vi "Teleop.vi"(10 "Match Info":T2={"Autonomous Elapsed Seconds"=0.0, "TeleOp Elapsed Seconds"=0.0, "Disabled Elapsed Seconds"=0.0, "Visited Autonomous"=FALSE, "Visited TeleOp"=FALSE, "Visited Disabled"=FALSE, "Autonomous Settings"={"Autonomous Style"=enum."Independent", "VI Refnum"=refnum}}, 11 "Call Context":T3) -> ()   [LabVIEW 2015]
doc: "This VI is called for each TeleOp packet received from the DS where the robot is not disabled. It is often used to read from the joysticks and update I/O or to update setpoints for timed control loops. It should complete and return within 20 milliseconds or it may miss DS packets."
uses:
  <vilib>/Rock Robotics/WPI/DriverStation/WPI_DriverStationDerivedRobotMode.ctl
  <vilib>/Rock Robotics/WPI/DriverStation/WPI_DriverStationMatch Info.ctl
  <vilib>/Rock Robotics/WPI/Utilities/WPI_GetSetVariantRefNum.vi
  <vilib>/Rock Robotics/Network Tables/SD Write Boolean Array.vi
  <vilib>/Rock Robotics/Network Tables/SD Read Boolean.vi
  <vilib>/Rock Robotics/Network Tables/SD Read Number.vi
  Robot Global Data.vi
  <vilib>/addons/control/pid/pid.llb/PID (DBL).vi
  <vilib>/Rock Robotics/WPI/RobotDrive/WPI_RobotDriveMecanumDrive_Cartesian.vi
  <vilib>/addons/control/pid/NI_PID_pid.lvlib
panel:
  in  "UseGyro?":bool
  out "Gyro":T1(graph)
  out "Rotation Input":dbl(graph)
  out "Sample Slider 0":dbl(slide) scale=0.0..5.0
  out "Sample Boolean 1":bool
  out "Sample Boolean 0":bool
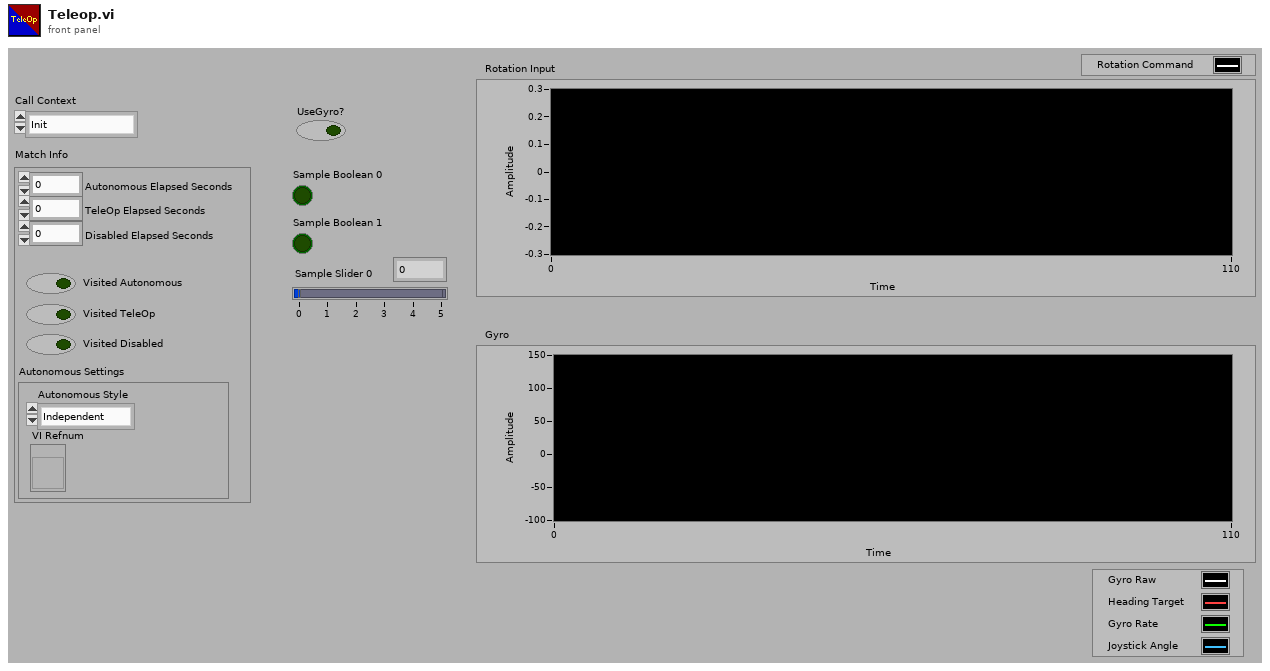
[diagram p1: front panel]
types:
  T1 = cluster{"Angle":dbl, "Heading":dbl, "Angular Rate":dbl, dbl}
  T2 = typedef "WPI_DriverStationMatch Info.ctl" = cluster{"Autonomous Elapsed Seconds":dbl, "TeleOp Elapsed Seconds":dbl, "Disabled Elapsed Seconds":dbl, "Visited Autonomous":bool, "Visited TeleOp":bool, "Visited Disabled":bool, "Autonomous Settings":cluster{"Autonomous Style":enum16{"Iterative", "Independent"}, "VI Refnum":refnum<vi>}}
  T3 = typedef "WPI_DriverStationDerivedRobotMode.ctl" = enum16{"Init", "Execute", "Stop"}
  T4 = cluster{"proportional gain (Kc)":dbl, "integral time (Ti, min)":dbl, "derivative time (Td, min)":dbl}
  T5 = typedef "WPI_JoystickDevRef.ctl" = cluster{"Device":T6}
  T6 = typedef "WPI_JoystickDeviceEnum.ctl" = enum16{"USB 0", "USB 1", "USB 2", "USB 3", "USB 4", "USB 5"}
  T7 = cluster{"Axes[0]":dbl, "Axes[1]":dbl, "Axes[2]":dbl, "Axes[3]":dbl, "Axes[4]":dbl, "Axes[5]":dbl, "Axes[6]":dbl, "Axes[7]":dbl, "Axes[8]":dbl}
  T8 = cluster{"Buttons[0]":bool, "Buttons[1]":bool, "Buttons[2]":bool, "Buttons[3]":bool, "Buttons[4]":bool, "Buttons[5]":bool, "Buttons[6]":bool, "Buttons[7]":bool, "Buttons[8]":bool}
  T9 = enum16{"CW_Fast", "CW_Slow", "CCW_Fast", "CCW_Slow", "Straight", "WaitingForStraight", "Rotate_Move"}
  T10 = cluster{"GyroHeading":dbl, "Heading":dbl, "GyroRate":dbl, dbl}
  T11 = typedef "WPI_RobotDriveDevRef.ctl" = cluster{"DevStatus":errorcluster, "Motors[]":T12[], "Square Inputs":bool, "Max Output":dbl}
  T12 = typedef "WPI_MotorControlDeviceRef.ctl" = cluster{"DeviceStatus":errorcluster, "Type":T13, "PWM":cluster{"PWM Channel":T14, "DeadBand":T15}, "CAN":cluster{"Device Number":u8, "Control Mode":T16, "Semaphore":T17, "Max Vout":dbl, "TalonSRX Control Mode":T18}, "Invert":bool}
  T13 = typedef "WPI_MotorControlType.ctl" = enum16{"PWM", "CAN", "CANTalonSRX"}
  T14 = typedef "FPGA_DIOPWMChannel.ctl" = enum8{"PWM 0", "PWM 1", "PWM 2", "PWM 3", "PWM 4", "PWM 5", "PWM 6", "PWM 7", "PWM 8", "PWM 9", "PWM MXP 0", "PWM MXP 1", "PWM MXP 2", "PWM MXP 3", "PWM MXP 4", "PWM MXP 5", "PWM MXP 6", "PWM MXP 7", "PWM MXP 8", "PWM MXP 9", "Invalid"}
  T15 = typedef "WPI_PWMDeadband.ctl" = cluster{"Name":string, "maxPositivePwm":i32, "minPositivePwm":i32, "centerPwm":i32, "maxNegativePwm":i32, "minNegativePwm":i32, "angularRange":u16}
  T16 = typedef "WPI_CANJaguar_ControlMode.ctl" = enum8{"Percent VBus", "Current", "Speed", "Position", "Voltage"}
  T17 = typedef "Semaphore RefNum" = refnum<k1>
  T18 = typedef "WPI_CANTalonSRX_APIControlMode.ctl" = enum8{"Percent VBus", "Speed", "Position", "Slave", "Unchanged / Invalid", "Voltage Compensation", "Current"}
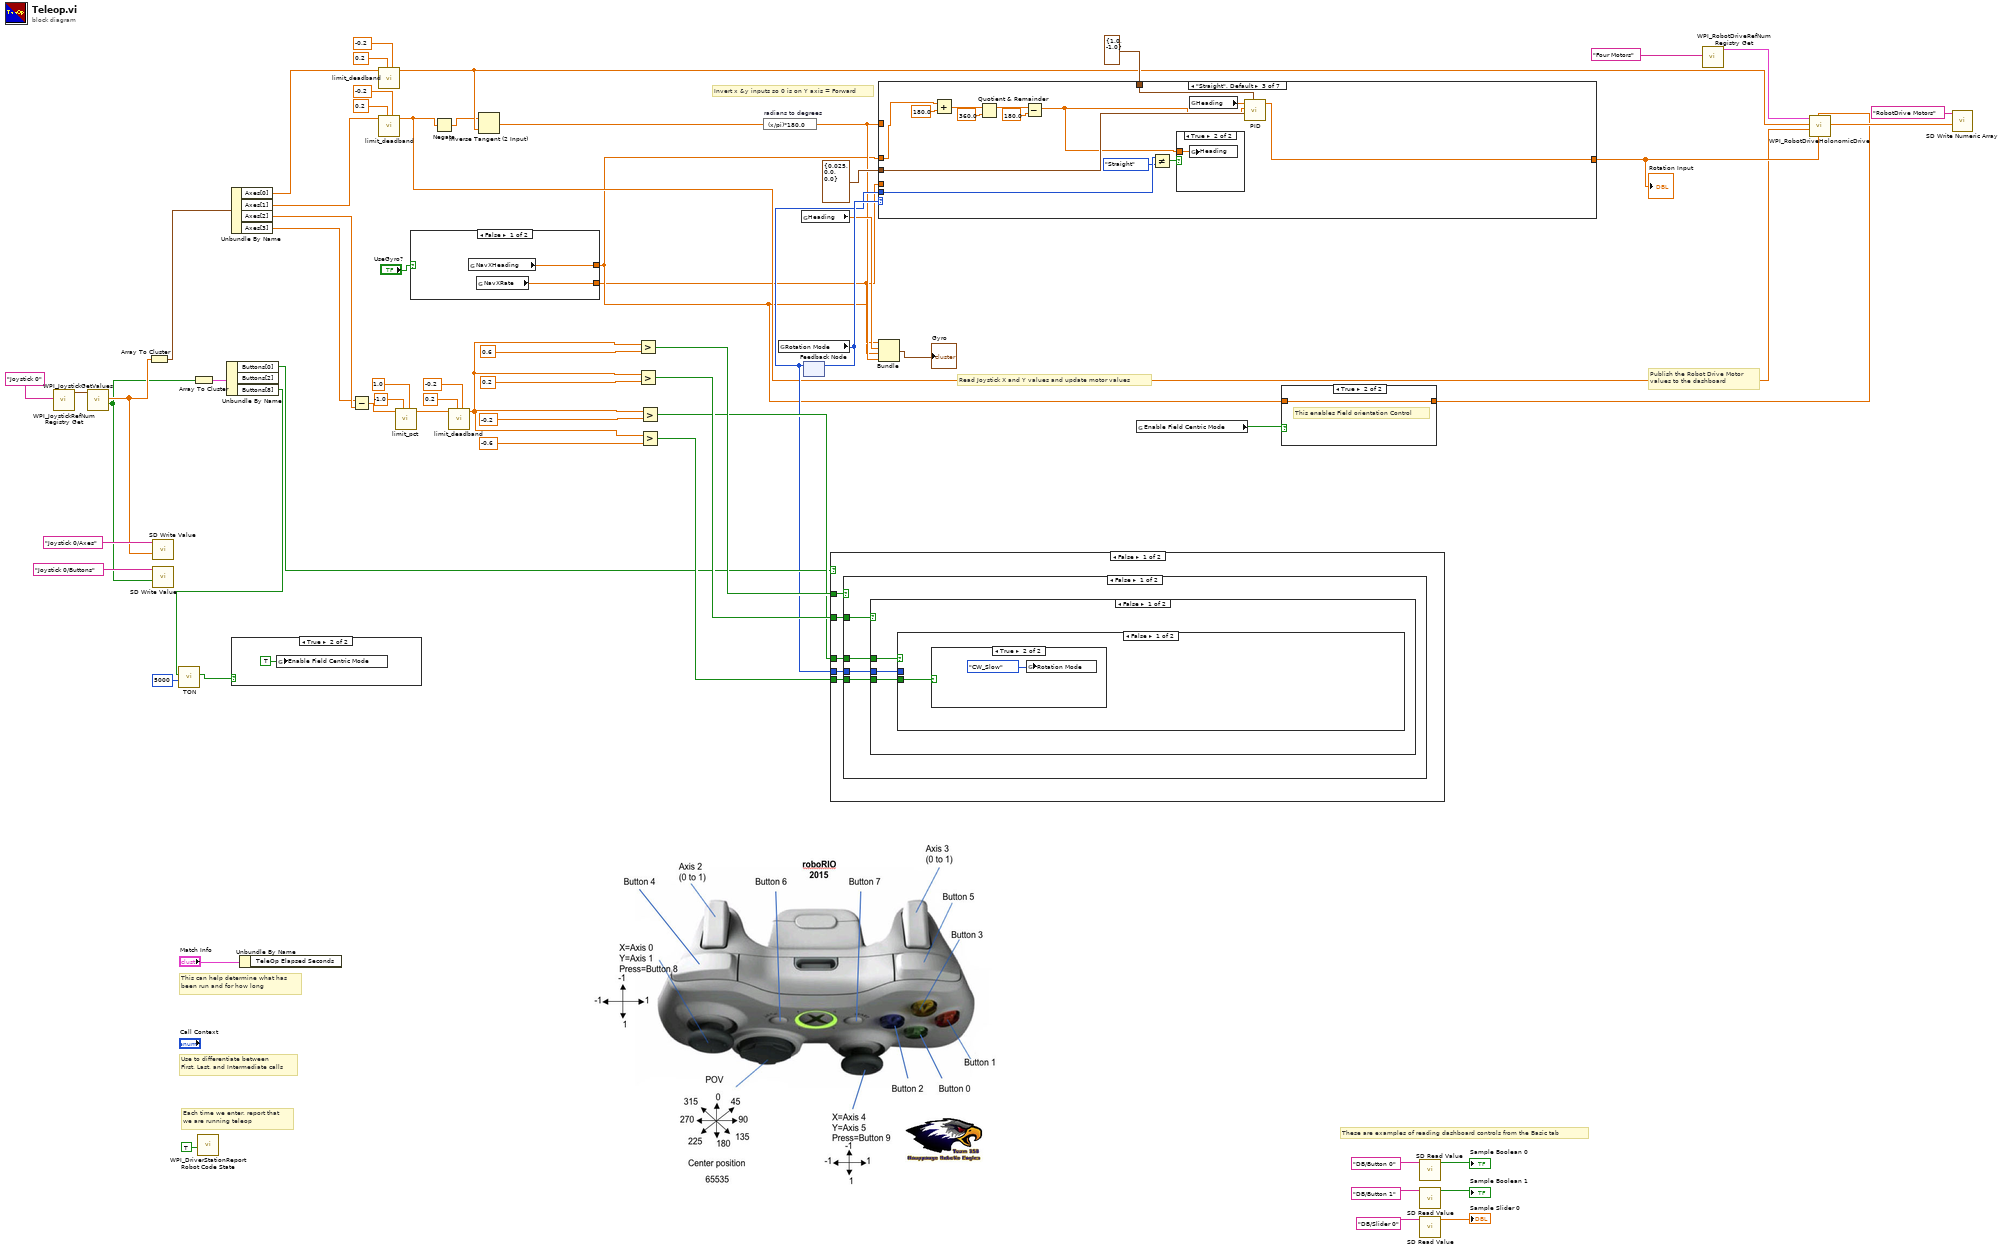
[diagram p0: block diagram]
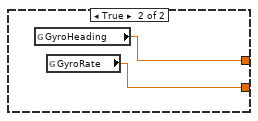
[diagram p2: hidden frame]
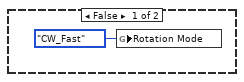
[diagram p4: hidden frame]
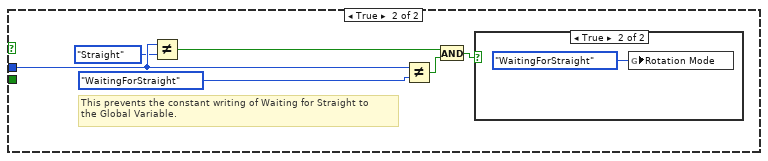
[diagram p5: hidden frame]
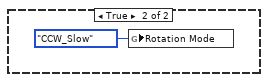
[diagram p7: hidden frame]
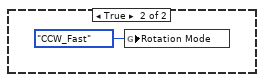
[diagram p8: hidden frame]
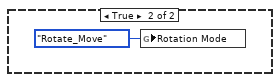
[diagram p9: hidden frame]
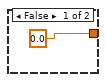
[diagram p10: hidden frame]
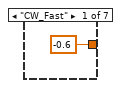
[diagram p11: hidden frame]
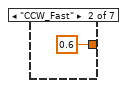
[diagram p12: hidden frame]
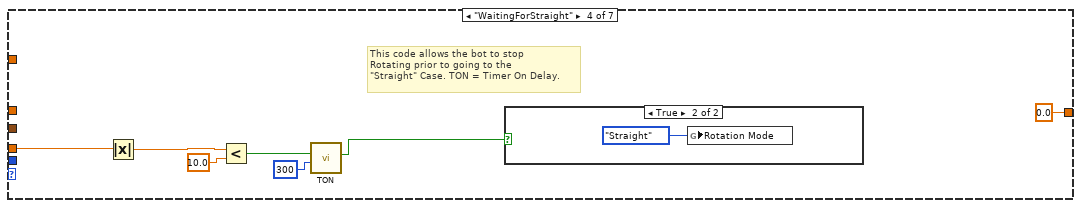
[diagram p14: hidden frame]
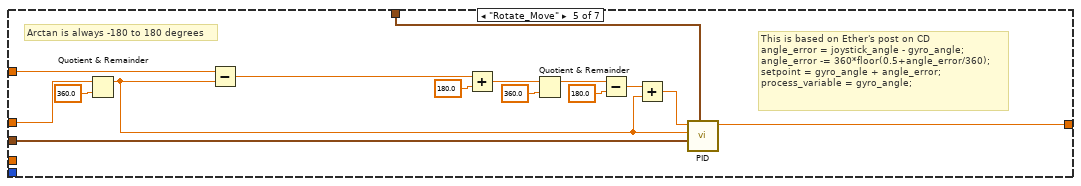
[diagram p16: hidden frame]
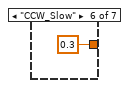
[diagram p17: hidden frame]
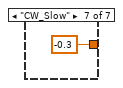
[diagram p18: hidden frame]
diagram:
  # "Invert x &y inputs so 0 is on Y axis = Forward"
  # "Publish the Robot Drive Motor\nvalues to the dashboard"
  # "Read Joystick X and Y values and update motor values"
  # "These are examples of reading dashboard controls from the Basic tab"
  # "Each time we enter, report that\nwe are running teleop"
  # "Use to differentiate between\nFirst, Last, and Intermediate calls"
  # "This can help determine what has\nbeen run and for how long"
  n1 = call <vilib>:"WPI_JoystickRefNum Registry Get.vi"("refnum name"="Joystick 0") -> ("JoystickDevRef"=w62:T5)  [unwired: 1 in, 9 out]
  n2 = call <vilib>:"WPI_JoystickGetValues.vi"("JoystickDevRef"=w62) -> ("Buttons"=w8:bool[], "Axes"=w10:dbl[])  [unwired: 6 in, 3 out]
  n3 = Array To Cluster(array=w10) -> (cluster=w9:T7)
  n4 = call-poly <vilib>:"SD Write Value.vi"("Numeric Array"=w10, "Name"="Joystick 0/Axes") -> ()  [unwired: 8 in, 2 out]
  n5 = call-poly <vilib>:"SD Write Value.vi"("Boolean Array"=w8, "Name"="Joystick 0/Buttons") -> ()  [unwired: 8 in, 2 out]
  n6 = Array To Cluster(array=w8) -> (cluster=w7:T8)
  n7 = call <vilib>:"WPI_DriverStationReport Robot Code State.vi"("TeleOp"=TRUE ("Autonomous")) -> ()  [unwired: 10 in, 1 out]
  n8 = Unbundle By Name(w7) -> ("Buttons[0]"=w29:bool, "Buttons[8]"=w2:bool)  [unwired: 1 out]
  n9 = call "TON.vi"("Delay (ms)"=u32 5000, "Input"=w2) -> ("Output"=w3:bool)  [unwired: 9 in]
  n10 = Unbundle By Name(w9) -> ("Axes[0]"=w28:dbl, "Axes[1]"=w16:dbl, "Axes[2]"=w19:dbl, "Axes[3]"=w18:dbl)
  n11 = case shown="True" w3 {
    frame False {
    }
    frame True {
      n12 = global write "Robot Global Data.vi" "Enable Field Centric Mode"(TRUE ("Enable Field Centric Mode")) -> ()
    }
  }
  n13 = Unbundle By Name("Match Info") -> ()  [unwired: 1 out]
  n14 = Subtract(x=w18, y=w19) -> (x-y=w20:dbl)
  n15 = call "limit_deadband.vi"("lower limit"=-0.2, "upper limit"=0.2, "Val"=w28) -> ("Val Out"=w14:dbl)  [unwired: 8 in]
  n16 = call "limit_deadband.vi"("lower limit"=-0.2, "upper limit"=0.2, "Val"=w16) -> ("Val Out"=w15:dbl)  [unwired: 8 in]
  n17 = call "limit_pct.vi"("upper limit"=1.0, "lower limit"=-1.0, "PCT"=w20) -> ("PCT Out"=w40:dbl)  [unwired: 8 in]
  n18 = case shown="False" "UseGyro?" {
    tunnel: [w67 w69] -> w5
    tunnel: [w66 w68] -> w4
    frame False {
      n19 = global read "Robot Global Data.vi" "NavXHeading"() -> (w67:dbl)
      n20 = global read "Robot Global Data.vi" "NavXRate"() -> (w66:dbl)
    }
    frame True {
      n21 = global read "Robot Global Data.vi" "GyroHeading"() -> (w69:dbl)
      n22 = global read "Robot Global Data.vi" "GyroRate"() -> (w68:dbl)
    }
  }
  n23 = Negate(x=w15) -> (-x=w13:dbl)
  n24 = call "limit_deadband.vi"("lower limit"=-0.2, "upper limit"=0.2, "Val"=w40) -> ("Val Out"=w33:dbl)  [unwired: 8 in]
  n25 = Inverse Tangent (2 Input)(1:w14, 2:w13) -> (0:w11:dbl)
  n26 = Greater?(x=w33, y=0.6 ("x")) -> (0:w39:bool)
  n27 = Greater?(x=w33, y=0.2 ("x")) -> (0:w38:bool)
  n28 = Greater?(x=w33, y=-0.2) -> (0:w34:bool)
  n29 = Greater?(x=w33, y=-0.6) -> (0:w31:bool)
  n30 = expression code="(x/pi)*180.0" "radians to degrees"(w11) -> (w12:dbl)
  n31 = global read "Robot Global Data.vi" "Rotation Mode"() -> (w25:T9)
  n32 = global read "Robot Global Data.vi" "Heading"() -> (w23:dbl)
  n33 = feedback #1() -> (w22:T9)  [unwired: 1 in]
  n34 = feedback-in #1(w25) -> ()
  n35 = case shown="False" w29 {
    tunnel: w39 -> [w74 _]
    tunnel: w38 -> [w73 _]
    tunnel: w34 -> [w72 _]
    tunnel: w31 -> [w71 _]
    tunnel: w22 -> [w70 _]
    frame False {
      n36 = case shown="False" w74 {
        tunnel: w73 -> [w78 _]
        tunnel: w72 -> [w77 _]
        tunnel: w71 -> [w76 _]
        tunnel: w70 -> [w75 _]
        frame False {
          n37 = case shown="False" w78 {
            tunnel: w77 -> [w81 _]
            tunnel: w76 -> [w80 _]
            tunnel: w75 -> [w79 _]
            frame False {
              n38 = case shown="False" w81 {
                tunnel: w80 -> [w82 _]
                tunnel: w79 -> [_ w90]
                frame False {
                  n39 = case shown="True" w82 {
                    frame False {
                      n40 = global write "Robot Global Data.vi" "Rotation Mode"(T9."CW_Fast" ("Rotation Mode")) -> ()
                    }
                    frame True {
                      n41 = global write "Robot Global Data.vi" "Rotation Mode"(T9."CW_Slow" ("Rotation Mode")) -> ()
                    }
                  }
                }
                frame True {
                  # "This prevents the constant writing of Waiting for Straight to \nthe Global Variable."
                  n42 = Not Equal?(x=w90, y=T9."Straight") -> (x != y?=w86:bool)
                  n43 = Not Equal?(x=w90, y=T9."WaitingForStraight") -> (x != y?=w85:bool)
                  n44 = And(x=w86, y=w85) -> (x .and. y?=w87:bool)
                  n45 = case shown="True" w87 {
                    frame False {
                    }
                    frame True {
                      n46 = global write "Robot Global Data.vi" "Rotation Mode"(T9."WaitingForStraight" ("Rotation Mode")) -> ()
                    }
                  }
                }
              }
            }
            frame True {
              n47 = global write "Robot Global Data.vi" "Rotation Mode"(T9."CCW_Slow" ("Rotation Mode")) -> ()
            }
          }
        }
        frame True {
          n48 = global write "Robot Global Data.vi" "Rotation Mode"(T9."CCW_Fast" ("Rotation Mode")) -> ()
        }
      }
    }
    frame True {
      n49 = global write "Robot Global Data.vi" "Rotation Mode"(T9."Rotate_Move" ("Rotation Mode")) -> ()
    }
  }
  n50 = case shown="\"Straight\", Default" w25 {
    tunnel: [-0.6 ("Rotation") 0.6 ("Rotation") w104 0.0 ("Rotation") w134 0.3 ("Rotation") -0.3 ("Rotation")] -> w24
    tunnel: w5 -> [_ _ w98 _ w121 _ _]
    tunnel: w4 -> [_ _ _ w113 _ _ _]
    tunnel: T4 {"proportional gain (Kc)"=0.025, "integral time (Ti, min)"=0.0, "derivative time (Td, min)"=0.0} ("PID gains") -> [_ _ w105 _ w133 _ _]
    tunnel: w12 -> [_ _ _ _ w127 _ _]
    tunnel: cluster{"output high":dbl, "output low":dbl} {"output high"=1.0, "output low"=-1.0} ("output range") -> [_ _ w106 _ w130 _ _]
    tunnel: w22 -> [_ _ w110 _ _ _ _]
    frame "CW_Fast" {
    }
    frame "CCW_Fast" {
    }
    frame "Straight", Default {
      n51 = Add(x=w98, y=180.0) -> (x+y=w101:dbl)
      n52 = Quotient & Remainder(x=w101, y=360.0) -> (x-y*floor(x/y)=w100:dbl)  [unwired: 1 out]
      n53 = Subtract(x=w100, y=180.0) -> (x-y=w97:dbl)
      n54 = Not Equal?(x=w110, y=T9."Straight" ("Rotation Mode")) -> (x != y?=w107:bool)
      n55 = case shown="True" w107 {
        tunnel: w97 -> [_ w111]
        frame False {
        }
        frame True {
          n56 = global write "Robot Global Data.vi" "Heading"(w111) -> ()
        }
      }
      n57 = global read "Robot Global Data.vi" "Heading"() -> (w108:dbl)
      n58 = call-poly <vilib>:"PID.vi"("output range"=w106, "PID gains"=w105, "process variable"=w97, "setpoint"=w108) -> ("output"=w104:dbl)  [unwired: 6 in, 1 out]
    }
    frame "WaitingForStraight" {
      # "This code allows the bot to stop \nRotating prior to going to the \n\"Straight\" Case. TON = Timer On Delay."
      n59 = Absolute Value(x=w113) -> (abs(x)=w112:dbl)
      n60 = Less?(x=w112, y=10.0) -> (x < y?=w115:bool)
      n61 = call "TON.vi"("Delay (ms)"=u32 300, "Input"=w115) -> ("Output"=w116:bool)  [unwired: 9 in]
      n62 = case shown="True" w116 {
        frame False {
        }
        frame True {
          n63 = global write "Robot Global Data.vi" "Rotation Mode"(T9."Straight" ("Rotation Mode")) -> ()
        }
      }
    }
    frame "Rotate_Move" {
      # "Arctan is always -180 to 180 degrees"
      # "This is based on Ether's post on CD\nangle_error = joystick_angle - gyro_angle;\nangle_error -= 360*floor(0.5+angle_error/360);\nsetpoint = gyro_angle + angle_error;\nprocess_variable = gyro_angle;"
      n64 = Quotient & Remainder(x=w121, y=360.0) -> (x-y*floor(x/y)=w120:dbl)  [unwired: 1 out]
      n65 = Subtract(x=w127, y=w120) -> (x-y=w129:dbl)
      n66 = Add(x=w129, y=180.0) -> (x+y=w126:dbl)
      n67 = Quotient & Remainder(x=w126, y=360.0) -> (x-y*floor(x/y)=w125:dbl)  [unwired: 1 out]
      n68 = Subtract(x=w125, y=180.0) -> (x-y=w123:dbl)
      n69 = Add(x=w123, y=w120) -> (x+y=w122:dbl)
      n70 = call-poly <vilib>:"PID.vi"("output range"=w130, "PID gains"=w133, "process variable"=w120, "setpoint"=w122) -> ("output"=w134:dbl)  [unwired: 6 in, 1 out]
    }
    frame "CCW_Slow" {
    }
    frame "CW_Slow" {
    }
  }
  "Rotation Input" <- w24
  n71 = Bundle("GyroHeading"=w5, "Heading"=w23, "GyroRate"=w4, w12) -> (→"Gyro":T10)  [unwired: 1 in]
  n72 = global read "Robot Global Data.vi" "Enable Field Centric Mode"() -> (w17:bool)
  n73 = case shown="True" w17 {
    tunnel: w5 -> [_ w138]
    tunnel: [0.0 ("Angle") w138] -> w30
    frame False {
    }
    frame True {
      # "This enables Field orientation Control"
    }
  }
  n74 = call-poly <vilib>:"SD Read Value.vi"("Name"="DB/Button 0" ("refnum name")) -> ("Boolean"=→"Sample Boolean 0":bool)  [unwired: 8 in, 2 out]
  n75 = call-poly <vilib>:"SD Read Value.vi"("Name"="DB/Button 1" ("refnum name")) -> ("Boolean"=→"Sample Boolean 1":bool)  [unwired: 8 in, 2 out]
  n76 = call-poly <vilib>:"SD Read Value.vi"("Name"="DB/Slider 0" ("refnum name")) -> ("Numeric"=→"Sample Slider 0":dbl)  [unwired: 8 in, 2 out]
  n77 = call <vilib>:"WPI_RobotDriveRefNum Registry Get.vi"("refnum name"="Four Motors") -> ("RobotDriveDevRef"=w51:T11)  [unwired: 1 in, 9 out]
  n78 = call-poly <vilib>:"WPI_RobotDriveHolonomicDrive.vi"("Rotation"=w24, "Gyro Angle"=w30, "Y"=w15, "X"=w14, "RobotDriveDevRef"=w51) -> ("Motor Values"=w49:dbl[])  [unwired: 4 in, 2 out]
  n79 = call <vilib>:"SD Write Numeric Array.vi"("Numeric Array"=w49, "Name"="RobotDrive Motors") -> ()  [unwired: 8 in, 2 out]
